vi "ErrorCaseStructure.vi"() -> ()   [LabVIEW 2014]
doc: "Use this template to create an application that executes until you click the Stop button. Unlike the Single Loop Application VI that uses polling, this VI uses the Event Structure."
panel:
  out "Error Out":errorcluster
  in  "Error In":errorcluster
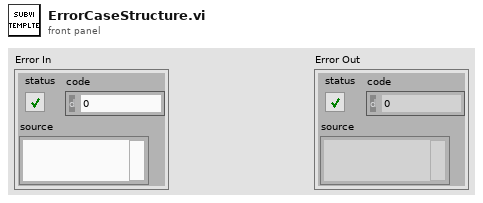
[diagram p1: front panel]
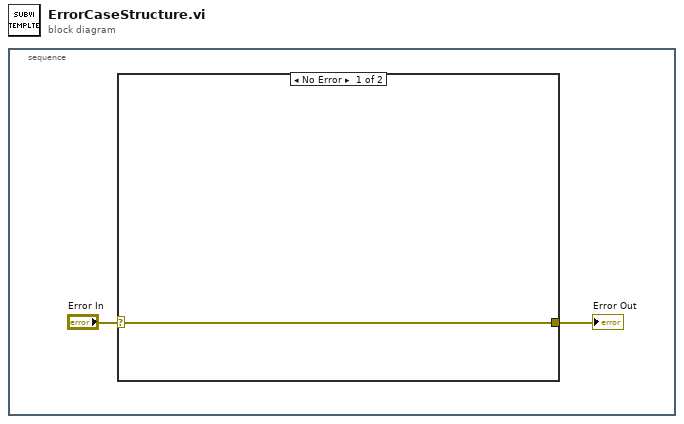
[diagram p0: block diagram]
diagram:
  n1 = stacked-sequence {
    frame #0 {
      n2 = case shown="No Error" "Error In" {
        selector: "Error In" -> [w3 w4]
        tunnel: [w3 w4] -> w1
        frame No Error {
        }
        frame Error {
        }
      }
      "Error Out" <- w1
    }
  }
